vi "Init Bfr Rx - Create Channels.vi"(5 "External Buffer":bool, 7 "Packet Name":string, 8 "error in (no error)":errorcluster, 11 "Data Access":refnum<class "Data Access Engine.lvclass">) -> (0 "error out":errorcluster, 3 "Buffered Receive Channels":T1)   [LabVIEW 2016, in "UDP-Custom-Device Engine.lvlib"]
uses:
  UDP-Custom-Device Engine.lvlib
  Types/Engine - Buffered Rx Channel Refs.ctl
  <vilib>/NI/NIVS Inline Async API/_Data Access Engine/Data Access Engine/Types/Write.DVR.ctl
  <vilib>/NI/NIVS Inline Async API/_Data Access Engine/Access Type Classes/Write/Write.lvclass
  <vilib>/NI/NIVS Inline Async API/_Data Access Engine/Data Access Engine/Types/Read.DVR.ctl
  <vilib>/NI/NIVS Inline Async API/_Data Access Engine/Access Type Classes/Read/Read.lvclass
  <vilib>/NI/NIVS Inline Async API/_Data Access Engine/Data Access Engine/Data Access Engine.lvclass
  <vilib>/NI/NIVS Inline Async API/_Data Access Engine/Data Access Engine/Methods/Read.Lookup.vi
  <vilib>/NI/NIVS Inline Async API/_Data Access Engine/Data Access Engine/Methods/Write.Lookup.vi
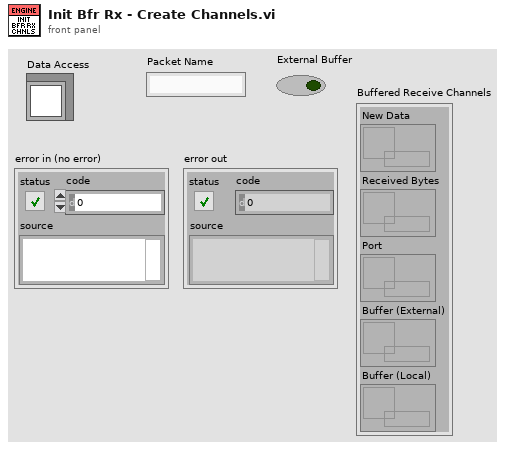
[diagram p1: front panel]
types:
  T1 = typedef "UDP-Custom-Device Engine.lvlib/Engine - Buffered Rx Channel Refs.ctl" = cluster{"New Data":T2, "Received Bytes":T2, "Port":T2, "Buffer (External)":T3, "Buffer (Local)":T2}
  T2 = typedef "Data Access Engine.lvlib/Data Access Engine.lvclass/Write.DVR.ctl" = refnum<data-value>
  T3 = typedef "Data Access Engine.lvlib/Data Access Engine.lvclass/Read.DVR.ctl" = refnum<data-value>
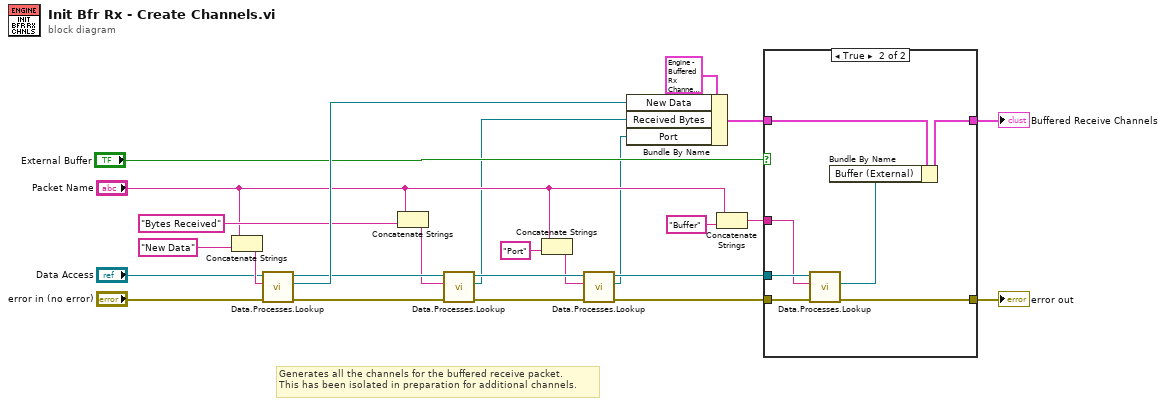
[diagram p0: block diagram]
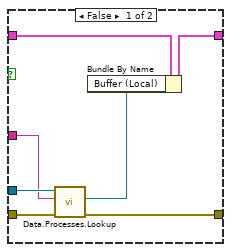
[diagram p2: hidden frame]
diagram:
  # "Generates all the channels for the buffered receive packet.\nThis has been isolated in preparation for additional channels."
  n1 = Concatenate Strings("Packet Name", "New Data" ("Item GUID")) -> (w25:string)
  n2 = call-poly <vilib>:"Data.Processes.Lookup.vi"("error in (no error)"="error in (no error)", "Name"=w25, "Data Access API in"="Data Access") -> ("error out"=w17:errorcluster, "Ref"=w20:T2, "Data Access API out"=w11:refnum<class "Data Access Engine.lvclass">)  [unwired: 5 in, 1 out]
  n3 = Concatenate Strings("Packet Name", "Bytes Received" ("string")) -> (w4:string)
  n4 = call-poly <vilib>:"Data.Processes.Lookup.vi"("error in (no error)"=w17, "Name"=w4, "Data Access API in"=w11) -> ("error out"=w16:errorcluster, "Ref"=w3:T2, "Data Access API out"=w10:refnum<class "Data Access Engine.lvclass">)  [unwired: 5 in, 1 out]
  n5 = Concatenate Strings("Packet Name", "Port" ("Item GUID")) -> (w6:string)
  n6 = call-poly <vilib>:"Data.Processes.Lookup.vi"("error in (no error)"=w16, "Name"=w6, "Data Access API in"=w10) -> ("error out"=w15:errorcluster, "Ref"=w5:T2, "Data Access API out"=w9:refnum<class "Data Access Engine.lvclass">)  [unwired: 5 in, 1 out]
  n7 = Bundle By Name(cluster=T1 {"New Data"=refnum, "Received Bytes"=refnum, "Port"=refnum, "Buffer (External)"=refnum, "Buffer (Local)"=refnum} ("Buffered Receive Channels"), "New Data"=w20, "Received Bytes"=w3, "Port"=w5) -> (w18:T1)
  n8 = Concatenate Strings("Packet Name", "Buffer" ("Item GUID")) -> (w8:string)
  n9 = case shown="True" "External Buffer" {
    tunnel: [w28 w35] -> w2
    tunnel: w18 -> [w29 w36]
    tunnel: [w26 w33] -> w1
    tunnel: w15 -> [w27 w34]
    tunnel: w9 -> [w32 w39]
    tunnel: w8 -> [w31 w38]
    frame False {
      n10 = call-poly <vilib>:"Data.Processes.Lookup.vi"("error in (no error)"=w27, "Name"=w31, "Data Access API in"=w32) -> ("error out"=w26:errorcluster, "Ref"=w30:T2)  [unwired: 5 in, 2 out]
      n11 = Bundle By Name(cluster=w29, "Buffer (Local)"=w30) -> (w28:T1)
    }
    frame True {
      n12 = call-poly <vilib>:"Data.Processes.Lookup.vi"("error in (no error)"=w34, "Name"=w38, "Data Access API in"=w39) -> ("error out"=w33:errorcluster, "Ref"=w37:T3)  [unwired: 5 in, 2 out]
      n13 = Bundle By Name(cluster=w36, "Buffer (External)"=w37) -> (w35:T1)
    }
  }
  "error out" <- w1
  "Buffered Receive Channels" <- w2
